vi "DAQ_OPC UA.vi"() -> (0 "Error Out":errorcluster)   [LabVIEW 2017]
uses:
  DAQmx Fill In Error Info.vi
  XDataNode.xnode
  C:/Program Files (x86)/National Instruments/LabVIEW 2017/resource/objmgr/ni.dex.rc
panel:
  out "Producer Loop Time":i64
  out "Consumer Loop Time":u32
  out "Time":dbl
  out "Available Elements for Writing":i32
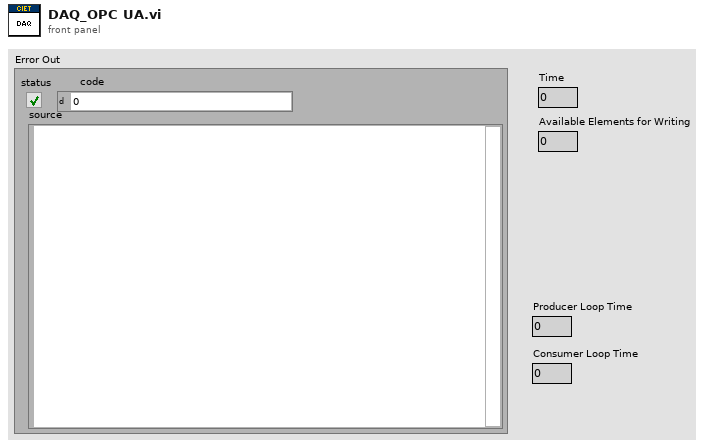
[diagram p1: front panel]
types:
  T1 = cluster{"Expected End [f-1]":u64, "Actual End [f-1]":u64, "Finished Late? [f-1]":bool, "Expected End [i-1]":u64, "Actual End [i-1]":u64, "Finished Late? [i-1]":bool, "Expected Start [i]":u64, "Actual Start [i]":u64, "Expected Start [f]":u64, "Actual Start [f]":u64, "Source Name":string, "Structure Name":string, "Period":i64, "Deadline":i64, "Offset":i64, "Start":i64, "Priority":i32, "Timeout":i32, "Mode":enum32{"No Change", "Process missed periods, maintain original phase", "Discard missed periods, maintain original phase", "Process missed periods, ignore original phase", "Discard missed periods, ignore original phase"}, "Wakeup Reason":enum32{"Normal", "Aborted", "Asynchronous wakeup", "Timing source error", "Timed loop error", "Timeout"}, "Error":errorcluster, "Source Type":string, "Secondary Source Type":string, "Global End Time":u64, "Global Start Time":u64, "Frame Duration":u64, "Iteration Duration":u64, "Assigned CPU":i32, "I/O Scan Engine Mode":u32}
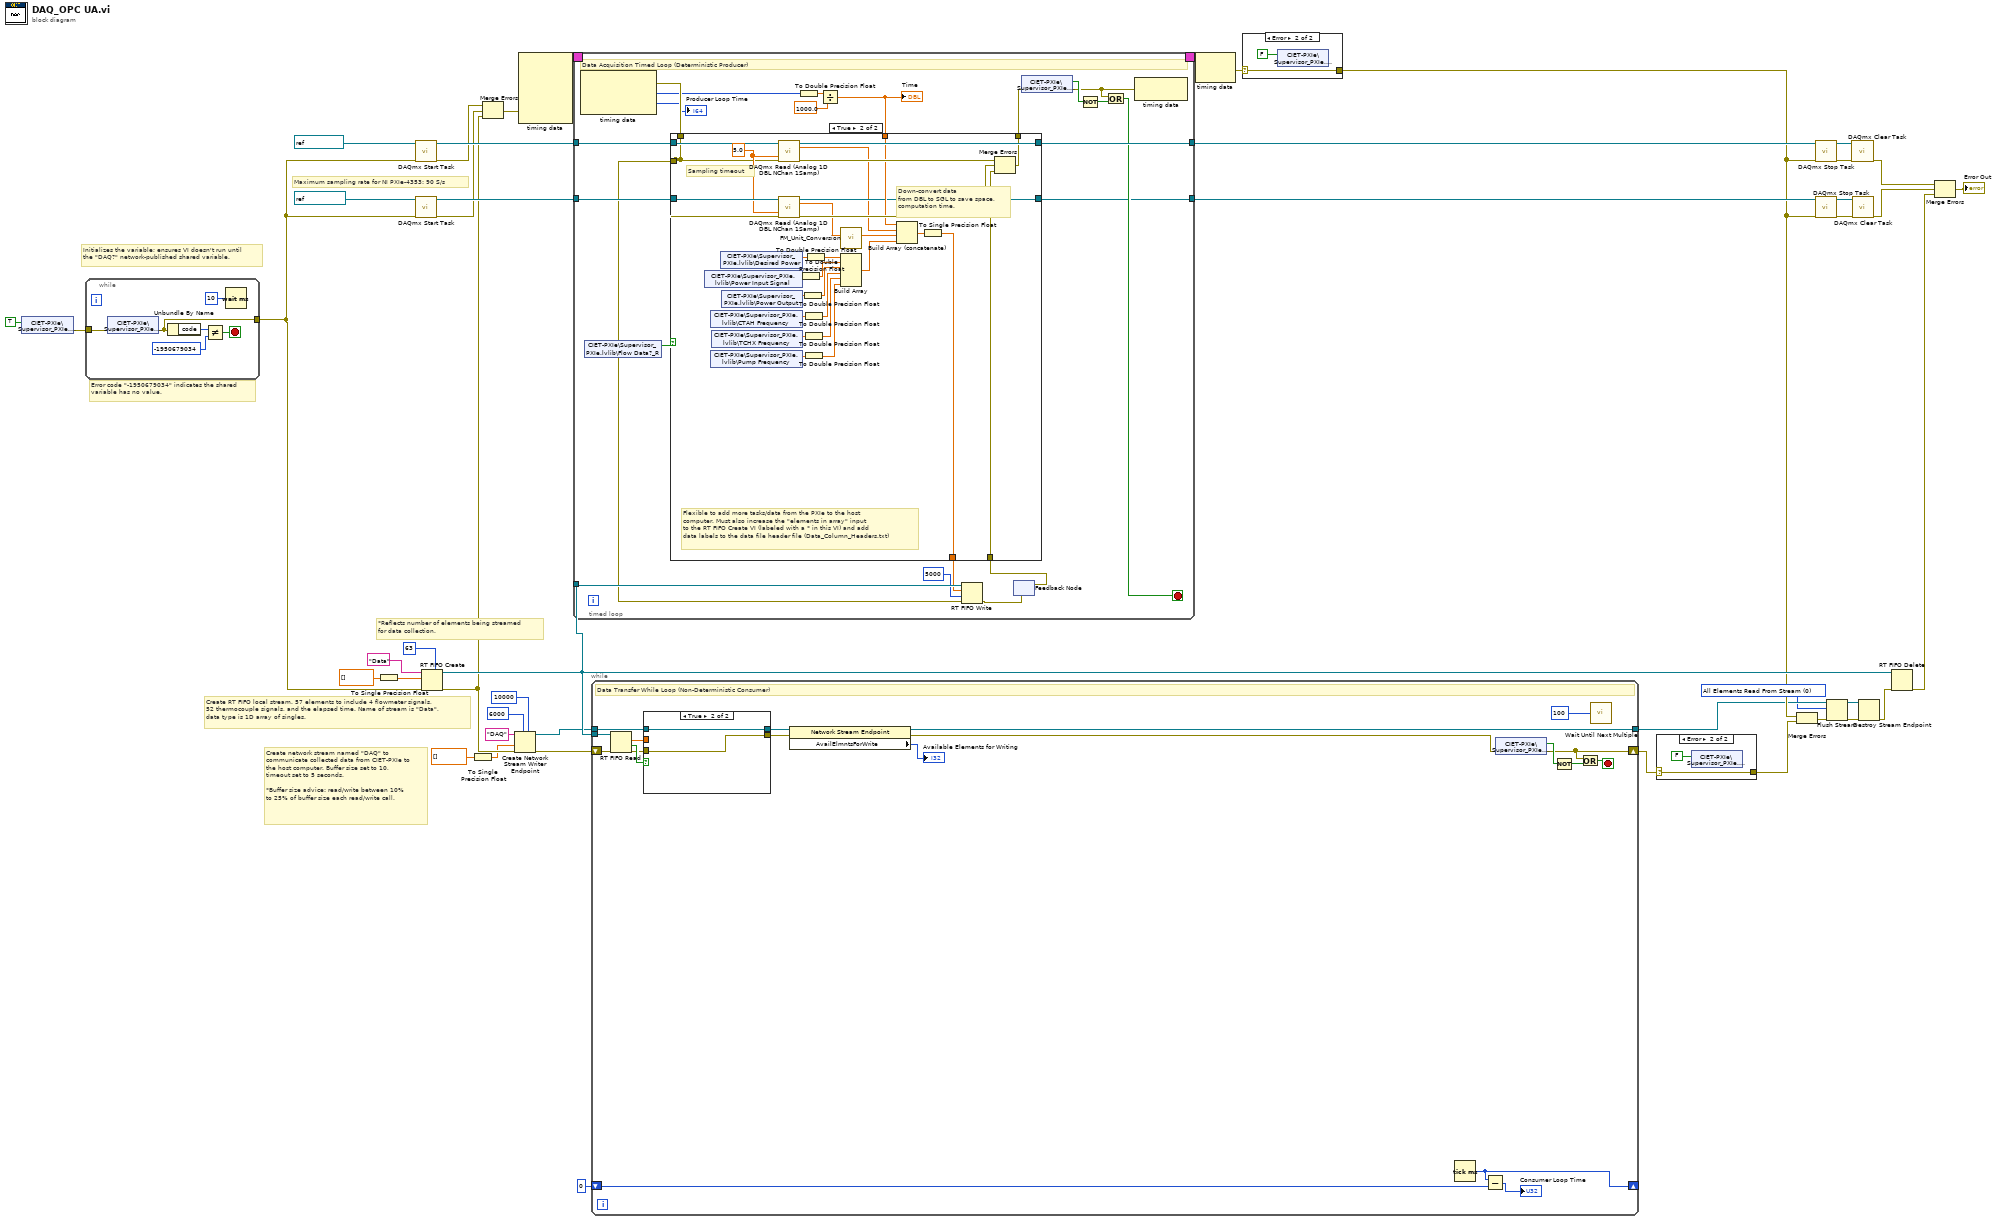
[diagram p0: block diagram]
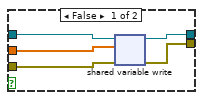
[diagram p4: hidden frame]
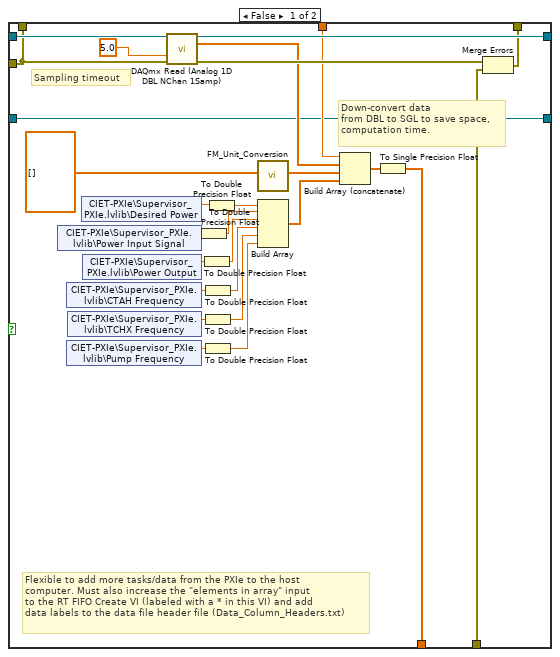
[diagram p5: hidden frame]
diagram:
  w2 = u8 0 items=["All Elements Read From Stream", "All Elements Available for Reading"] ("wait condition")
  # "*Reflects number of elements being streamed\nfor data collection."
  # "Create RT FIFO local stream. 57 elements to include 4 flowmeter signals,\n52 thermocouple signals, and the elapsed time. Name of stream is \"Data\",\ndata type is 1D array of singles."
  # "Create network stream named \"DAQ\" to communicate collected data from CIET-PXIe to the host computer. Buffer size set to 10, timeout set to 5 seconds. \n\n*Buffer size advice: read/write between 10%\nto 25% of buffer size each read/write call."
  # "Maximum sampling rate for NI PXIe-4353: 90 S/s"
  # "Initializes the variable; ensures VI doesn't run until\nthe \"DAQ?\" network-published shared variable."
  # "Error code \"-1950679034\" indicates the shared\nvariable has no value."
  n1 = shared-variable "CIET-PXIe\\Supervisor_PXIe.lvlib\\DAQ?"(TRUE ("Active?")) -> (error out=w22:errorcluster)  [unwired: 1 in]
  n2 = while {
    tunnel: w22 -> [w51]
    tunnel: [w50] -> w21
    stop <- w47 stop-if-true
    n3 = shared-variable "CIET-PXIe\\Supervisor_PXIe.lvlib\\DAQ?"(error in=w51) -> (error out=w50:errorcluster)  [unwired: 1 out]
    n4 = Unbundle By Name(w50) -> ("code"=w49:i32)
    n5 = Not Equal?(x=w49, y=-1950679034) -> (x != y?=w47:bool)
    n6 = Wait (ms)(milliseconds to wait=u32 10) -> ()  [unwired: 1 out]
  }
  n7 = To Single Precision Float(number=dbl[] []) -> (single precision float=w32:sgl[])
  n8 = call "DAQmx Start Task.vi"("task/channels in"=refnum<k21> "CIET-TC", "error in"=w21) -> ("task out"=w42:refnum<k21>, "error out"=w26:errorcluster)  [unwired: 12 in]
  n9 = call "DAQmx Start Task.vi"("task/channels in"=refnum<k21> "CIET-FM", "error in"=w21) -> ("task out"=w41:refnum<k21>, "error out"=w27:errorcluster)  [unwired: 12 in]
  n10 = RT FIFO Create(0:"Data" ("name (unnamed)"), 1:w32, 3:w21, 6:u32 63 ("elements in array (1)")) -> (8:w25:refnum<k33>, 11:w17:errorcluster)  [unwired: 4 in, 1 out]
  n11 = To Single Precision Float(number=dbl[] []) -> (single precision float=w7:sgl[])
  n12 = Merge Errors(w26, w27, w17) -> (w28:errorcluster)
  n13 = Create Network Stream Writer Endpoint(5:10000 ("timeout in ms (-1)"), 7:6000 ("writer buffer size"), 8:w17, 9:w7, 11:"DAQ" ("writer name")) -> (0:w18:errorcluster, 3:w16:refnum<k21>)  [unwired: 2 in]
  n14 = node-c288(w28) -> (w46:T1)  [unwired: 4 in]
  n15 = timed-loop {
    timing: w46 -> [_]
    timing-out: [_] -> w45
    tunnel: w25 -> [w71]
    tunnel: w42 -> [w74]
    tunnel: [w72] -> w36
    tunnel: w41 -> [w73]
    tunnel: [w59] -> w35
    stop <- w66 stop-if-true
    # "Data Acquisition Timed Loop (Deterministic Producer)"
    n16 = node-c288() -> (w69:errorcluster, w60:i64, →"Producer Loop Time":i64)  [unwired: 1 in]
    n17 = shared-variable "CIET-PXIe\\Supervisor_PXIe.lvlib\\Flow Data?_R"() -> (w53:bool)  [unwired: 1 in, 1 out]
    n18 = To Double Precision Float(number=w60) -> (double precision float=w63:dbl)
    n19 = Divide(x=w63, y=1000.0) -> (x/y=w62:dbl)
    "Time" <- w62
    n20 = feedback #1() -> (w55:errorcluster)  [unwired: 1 in]
    n21 = case shown="True" w53 {
      tunnel: w74 -> [w101 w130]
      tunnel: w73 -> [w84 w129]
      tunnel: [w99 w127] -> w72
      tunnel: [w97 w125] -> w57
      tunnel: w69 -> [w81 w108]
      tunnel: w55 -> [w82 w122]
      tunnel: [w95 w121] -> w65
      tunnel: w62 -> [w94 w120]
      tunnel: [w84 w119] -> w59
      tunnel: [w81 w108] -> w54
      frame False {
        # "Flexible to add more tasks/data from the PXIe to the host \ncomputer. Must also increase the \"elements in array\" input \nto the RT FIFO Create VI (labeled with a * in this VI) and add\ndata labels to the data file header file (Data_Column_Headers.txt)"
        # "Down-convert data\nfrom DBL to SGL to save space,\ncomputation time."
        # "Sampling timeout"
        n22 = shared-variable "CIET-PXIe\\Supervisor_PXIe.lvlib\\Power Input Signal"() -> (w79:sgl)  [unwired: 1 in, 1 out]
        n23 = shared-variable "CIET-PXIe\\Supervisor_PXIe.lvlib\\CTAH Frequency"() -> (w86:sgl)  [unwired: 1 in, 1 out]
        n24 = shared-variable "CIET-PXIe\\Supervisor_PXIe.lvlib\\Pump Frequency"() -> (w88:sgl)  [unwired: 1 in, 1 out]
        n25 = shared-variable "CIET-PXIe\\Supervisor_PXIe.lvlib\\TCHX Frequency"() -> (w87:sgl)  [unwired: 1 in, 1 out]
        n26 = shared-variable "CIET-PXIe\\Supervisor_PXIe.lvlib\\Desired Power"() -> (w80:sgl)  [unwired: 1 in, 1 out]
        n27 = shared-variable "CIET-PXIe\\Supervisor_PXIe.lvlib\\Power Output"() -> (w78:sgl)  [unwired: 1 in, 1 out]
        n28 = call "DAQmx Read (Analog 1D DBL NChan 1Samp).vi"("task/channels in"=w101, "timeout"=5.0, "error in"=w81) -> ("task out"=w99:refnum<k21>, "data"=w93:dbl[], "error out"=w96:errorcluster)  [unwired: 10 in]
        n29 = To Double Precision Float(number=w79) -> (double precision float=w76:dbl)
        n30 = To Double Precision Float(number=w78) -> (double precision float=w75:dbl)
        n31 = To Double Precision Float(number=w86) -> (double precision float=w89:dbl)
        n32 = To Double Precision Float(number=w87) -> (double precision float=w90:dbl)
        n33 = To Double Precision Float(number=w88) -> (double precision float=w91:dbl)
        n34 = To Double Precision Float(number=w80) -> (double precision float=w77:dbl)
        n35 = call "FM_Unit_Conversion.vi"("Input Array [A]"=dbl[] []) -> ("Output Array [kg/h]"=w92:dbl[])  [unwired: 10 in]
        n36 = Build Array(w77, w76, w75, w89, w90, w91) -> (w85:dbl[])
        n37 = Build Array (concatenate)(w94, w93, w92, w85) -> (w98:dbl[])
        n38 = To Single Precision Float(number=w98) -> (single precision float=w97:sgl[])
        n39 = Merge Errors(w96, w82) -> (w95:errorcluster)
      }
      frame True {
        w128 = 5.0 ("timeout")
        # "Flexible to add more tasks/data from the PXIe to the host \ncomputer. Must also increase the \"elements in array\" input \nto the RT FIFO Create VI (labeled with a * in this VI) and add\ndata labels to the data file header file (Data_Column_Headers.txt)"
        # "Down-convert data\nfrom DBL to SGL to save space,\ncomputation time."
        # "Sampling timeout"
        n40 = shared-variable "CIET-PXIe\\Supervisor_PXIe.lvlib\\Power Input Signal"() -> (w105:sgl)  [unwired: 1 in, 1 out]
        n41 = shared-variable "CIET-PXIe\\Supervisor_PXIe.lvlib\\CTAH Frequency"() -> (w110:sgl)  [unwired: 1 in, 1 out]
        n42 = shared-variable "CIET-PXIe\\Supervisor_PXIe.lvlib\\Pump Frequency"() -> (w112:sgl)  [unwired: 1 in, 1 out]
        n43 = shared-variable "CIET-PXIe\\Supervisor_PXIe.lvlib\\TCHX Frequency"() -> (w111:sgl)  [unwired: 1 in, 1 out]
        n44 = shared-variable "CIET-PXIe\\Supervisor_PXIe.lvlib\\Desired Power"() -> (w107:sgl)  [unwired: 1 in, 1 out]
        n45 = shared-variable "CIET-PXIe\\Supervisor_PXIe.lvlib\\Power Output"() -> (w103:sgl)  [unwired: 1 in, 1 out]
        n46 = call "DAQmx Read (Analog 1D DBL NChan 1Samp).vi"("task/channels in"=w130, "timeout"=w128, "error in"=w108) -> ("task out"=w127:refnum<k21>, "data"=w118:dbl[], "error out"=w123:errorcluster)  [unwired: 10 in]
        n47 = call "DAQmx Read (Analog 1D DBL NChan 1Samp).vi"("task/channels in"=w129, "timeout"=w128, "error in"=w108) -> ("task out"=w119:refnum<k21>, "data"=w116:dbl[], "error out"=w124:errorcluster)  [unwired: 10 in]
        n48 = To Double Precision Float(number=w105) -> (double precision float=w104:dbl)
        n49 = To Double Precision Float(number=w103) -> (double precision float=w102:dbl)
        n50 = To Double Precision Float(number=w110) -> (double precision float=w113:dbl)
        n51 = To Double Precision Float(number=w111) -> (double precision float=w114:dbl)
        n52 = To Double Precision Float(number=w112) -> (double precision float=w115:dbl)
        n53 = To Double Precision Float(number=w107) -> (double precision float=w106:dbl)
        n54 = call "FM_Unit_Conversion.vi"("Input Array [A]"=w116) -> ("Output Array [kg/h]"=w117:dbl[])  [unwired: 10 in]
        n55 = Build Array(w106, w104, w102, w113, w114, w115) -> (w109:dbl[])
        n56 = Build Array (concatenate)(w120, w118, w117, w109) -> (w126:dbl[])
        n57 = To Single Precision Float(number=w126) -> (single precision float=w125:sgl[])
        n58 = Merge Errors(w123, w124, w122) -> (w121:errorcluster)
      }
    }
    n59 = RT FIFO Write(0:w71, 1:w57, 2:5000 ("timeout in ms (0)"), 3:w54) -> (11:w56:errorcluster)  [unwired: 1 in, 3 out]
    n60 = feedback-in #1(w56) -> ()
    n61 = shared-variable "CIET-PXIe\\Supervisor_PXIe.lvlib\\DAQ?"(error in=w65) -> (w68:bool, error out=w64:errorcluster)
    n62 = Not(x=w68) -> (.not. x?=w67:bool)
    n63 = Or(x=w64, y=w67) -> (x .or. y?=w66:bool)
    n64 = node-c288(w64) -> ()  [unwired: 1 out]
  }
  n65 = while {
    tunnel: w25 -> [w156]
    shift-right: [w145] -> w19
    shift-left: w18 -> [w155]
    tunnel: w16 -> [w147]
    tunnel: [w142] -> w9
    shift-right: [w140] -> _
    shift-left: u32 0 ("millisecond timer value") -> [w139]
    stop <- w148 stop-if-true
    # "Data Transfer While Loop (Non-Deterministic Consumer)"
    n66 = RT FIFO Read(0:w156, 3:w155) -> (9:w152:sgl[], 10:w153:bool, 11:w151:errorcluster)  [unwired: 2 in, 2 out]
    n67 = case shown="True" w153 {
      tunnel: w152 -> [w157 _]
      tunnel: w151 -> [w161 w163]
      tunnel: [w160 w163] -> w144
      tunnel: w147 -> [w159 w162]
      tunnel: [w158 w162] -> w143
      frame False {
        n68 = shared-variable-write(w159, w161, w157) -> (w158:refnum<k21>, w160:errorcluster)  [unwired: 1 in, 1 out]
      }
      frame True {
      }
    }
    n69 = property class="Network Stream Endpoint"(reference=w143, error in=w144) -> (reference out=w142:refnum<k21>, error out=w141:errorcluster, "AvailElmntsForWrite"=→"Available Elements for Writing":i32)
    n70 = Tick Count (ms)() -> (millisecond timer value=w140:u32)
    n71 = Subtract(x=w140, y=w139) -> (x-y=→"Consumer Loop Time":u32)
    n72 = shared-variable "CIET-PXIe\\Supervisor_PXIe.lvlib\\DAQ?"(error in=w141) -> (w150:bool, error out=w145:errorcluster)
    n73 = Not(x=w150) -> (.not. x?=w149:bool)
    n74 = Or(x=w145, y=w149) -> (x .or. y?=w148:bool)
    n75 = call "Wait Until Next Multiple"("Count(mSec)"=u32 100) -> ()  [unwired: 1 out]
  }
  n76 = node-c288(w45) -> (w20:errorcluster)
  n77 = case shown="Error" w20 {
    selector: w20 -> [w164 w165]
    tunnel: [w164 w165] -> w15
    frame No Error {
    }
    frame Error {
      n78 = shared-variable "CIET-PXIe\\Supervisor_PXIe.lvlib\\DAQ?"(FALSE ("DAQ?")) -> ()  [unwired: 1 in, 1 out]
    }
  }
  n79 = case shown="Error" w19 {
    selector: w19 -> [w167 w168]
    tunnel: [w167 w168] -> w14
    frame No Error {
    }
    frame Error {
      n80 = shared-variable "CIET-PXIe\\Supervisor_PXIe.lvlib\\DAQ?"(FALSE ("DAQ?")) -> ()  [unwired: 1 in, 1 out]
    }
  }
  n81 = Merge Errors(w15, w14) -> (w11:errorcluster)
  n82 = call "DAQmx Stop Task.vi"("task/channels in"=w36, "error in"=w15) -> ("task out"=w39:refnum<k21>, "error out"=w40:errorcluster)  [unwired: 12 in]
  n83 = call "DAQmx Stop Task.vi"("task/channels in"=w35, "error in"=w15) -> ("task out"=w37:refnum<k21>, "error out"=w38:errorcluster)  [unwired: 12 in]
  n84 = Flush Stream(8:w11, 10:w2, 11:w9) -> (0:w13:errorcluster, 3:w12:refnum<k21>)  [unwired: 1 in, 1 out]
  n85 = call "DAQmx Clear Task.vi"("task in"=w39, "error in"=w40) -> ("error out"=w34:errorcluster)  [unwired: 13 in]
  n86 = call "DAQmx Clear Task.vi"("task in"=w37, "error in"=w38) -> ("error out"=w33:errorcluster)  [unwired: 13 in]
  n87 = Destroy Stream Endpoint(8:w13, 11:w12) -> (0:w10:errorcluster)
  n88 = RT FIFO Delete(0:w25, 3:w10) -> (11:w4:errorcluster)  [unwired: 1 in]
  n89 = Merge Errors(w34, w33, w4) -> (→"Error Out":errorcluster)
